vi "catch.vi"(8 "error out":errorcluster, 11 "KNR out":T2) -> (0 "error out 2":errorcluster, 1 "Circles (Shape Detection 1)":T1(array[cluster]) {"Position"."Y" format="%.2f"; "Position"."X" format="%.2f"}, 2 "Number of Matches (Shape Detection 1)":i32, 3 "KNR out 2":T2, 10 "X":dbl)   [LabVIEW 2013]
uses:
  <userlib>/KNR OS 3.0 LabVIEW Toolkit/Type Definition/KNR3 Reference.ctl
  <userlib>/_FPGA Interface Advanced Tools/FPGA Interface Base/FPGA Interface Base.lvclass
  <userlib>/KNR OS 3.0 LabVIEW Toolkit/Type Definition/Resource.ctl
panel:
  out "Voltage":dbl
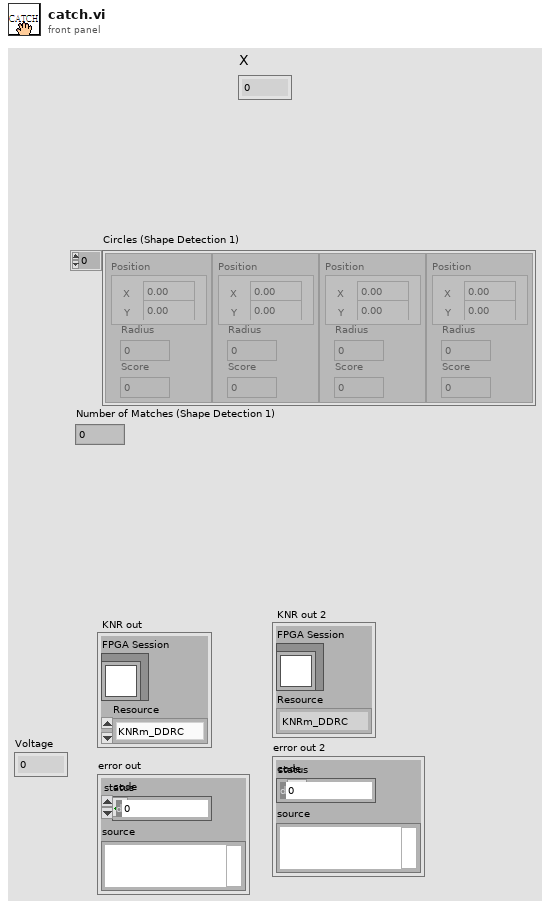
[diagram p1: front panel]
types:
  T1 = cluster{"Position":cluster{"X":sgl, "Y":sgl}, "Radius":dbl, "Score":dbl}[]
  T2 = typedef "KNR3 Reference.ctl" = cluster{"FPGA Session":refnum<class "FPGA Interface Base.lvclass">, "Resource":T3}
  T3 = typedef "Resource.ctl" = enum16{"KNRm_DDRC", "KNRm_DDDD", "KNRm_DDDR", "KNRm_DDDC", "KNR"}
  T4 = cluster{"Mode":enum16{"FRWD", "TURFIX", "TURNOF", "CIRCULAR"}, "Dir":enum16{"Left", "Right"}, "Pcmd":dbl, "Vcmd":dbl, "X":dbl, "Y":dbl}
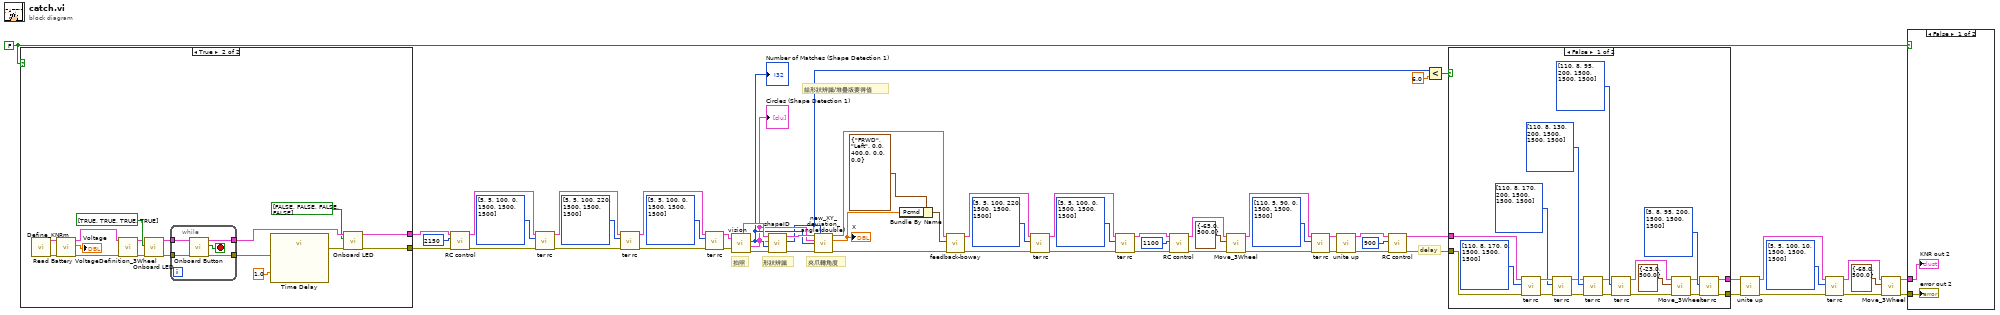
[diagram p0: block diagram]
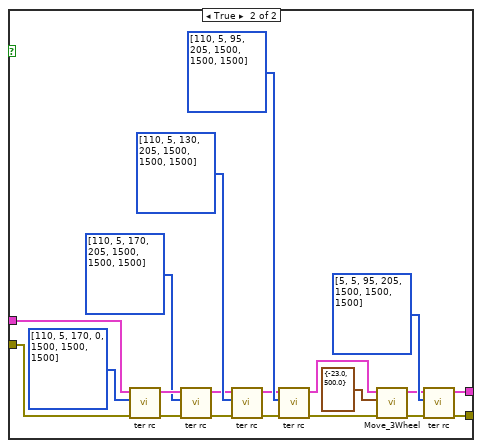
[diagram p2: hidden frame]
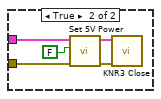
[diagram p3: hidden frame]
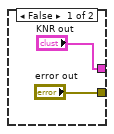
[diagram p4: hidden frame]
diagram:
  w61 = FALSE
  # "夾爪轉角度"
  # "形狀辨識"
  # "給形狀辨識/堆疊版要得值"
  # "拍照"
  # "delay"
  n1 = case shown="True" w61 {
    tunnel: ["KNR out" w69] -> w27
    tunnel: ["error out" w68] -> w26
    frame False {
    }
    frame True {
      n2 = call "Define_KNRm.vi"() -> ("error out"=w73:errorcluster, "KNR out"=w72:T2)  [unwired: 10 in]
      n3 = call <userlib>:"Read Battery Voltage.vi"("error in (no error)"=w73, "KNR in"=w72) -> ("error out"=w66:errorcluster, "Voltage"=→"Voltage":dbl, "KNR out"=w67:T2)  [unwired: 7 in]
      n4 = call "Definition_3Wheel.vi"("error in (no error)"=w66, "KNR in"=w67) -> ("error out"=w64:errorcluster, "KNR out"=w65:T2)  [unwired: 8 in]
      n5 = call <userlib>:"Onboard LED.vi"("error in (no error)"=w64, "LED List"=bool[] [TRUE, TRUE, TRUE, TRUE], "KNR in"=w65) -> ("error out"=w79:errorcluster, "KNR out"=w80:T2)  [unwired: 7 in]
      n6 = while {
        tunnel: w80 -> [w84]
        tunnel: w79 -> [w83]
        tunnel: [w82] -> w78
        tunnel: [w81] -> w76
        stop <- w85 stop-if-true
        n7 = call <userlib>:"Onboard Button.vi"("error in (no error)"=w83, "KNR in"=w84) -> ("error out"=w81:errorcluster, "value"=w85:bool, "KNR out"=w82:T2)  [unwired: 7 in]
      }
      n8 = call "Time Delay"("error in (no error)"=w76, "Delay Time (s)"=1.0) -> ("error out"=w75:errorcluster)  [unwired: 9 in]
      n9 = call <userlib>:"Onboard LED.vi"("error in (no error)"=w75, "LED List"=bool[] [FALSE, FALSE, FALSE, FALSE], "KNR in"=w78) -> ("error out"=w68:errorcluster, "KNR out"=w69:T2)  [unwired: 7 in]
    }
  }
  n10 = call "RC control.vi"("error in (no error)"=w26, "position"=2150, "KNR in"=w27) -> ("error out"=w50:errorcluster, "KNR out"=w51:T2)  [unwired: 7 in]
  n11 = call "ter rc.vi"("error in 2"=w50, "RC"=u16[] [5, 5, 100, 0, 1500, 1500, 1500], "KNR in 3"=w51) -> ("error out 4"=w34:errorcluster, "KNR out 4"=w35:T2)  [unwired: 7 in]
  n12 = call "ter rc.vi"("error in 2"=w34, "RC"=u16[] [5, 5, 100, 220, 1500, 1500, 1500], "KNR in 3"=w35) -> ("error out 4"=w23:errorcluster, "KNR out 4"=w47:T2)  [unwired: 7 in]
  n13 = call "ter rc.vi"("error in 2"=w23, "RC"=u16[] [5, 5, 100, 0, 1500, 1500, 1500], "KNR in 3"=w47) -> ("error out 4"=w55:errorcluster, "KNR out 4"=w56:T2)  [unwired: 7 in]
  n14 = call "vision.vi"("KNR in"=w56, "Error"=w55) -> ("KNR out"=w19:T2, "Number of Matches (Shape Detection 1)"=w15:i32, "Circles (Shape Detection 1)"=w14:T1, "error out"=w18:errorcluster)  [unwired: 1 in, 1 out]
  "Circles (Shape Detection 1)" <- w14
  "Number of Matches (Shape Detection 1)" <- w15
  n15 = call "shapeID.vi"("Error"=w18, "Nb Circles (Circle Detection 1)"=w15, "Circles (Shape Detection 1)"=w14, "KNR in"=w19) -> ("error out 4"=w16:errorcluster, "配對數"=w1:i32, "KNR out"=w17:T2)  [unwired: 4 in, 1 out]
  n16 = call "new_XY_deviation_angle(double).vi"("KNR in"=w17, "配對數"=w1, "Circles (Shape Detection 1)"=w14, "ふ计"=w15, "Error"=w16) -> ("KNR out"=w6:T2, "X"=w12:dbl, "error out"=w5:errorcluster)  [unwired: 6 in, 2 out]
  "X" <- w12
  n17 = Bundle By Name(cluster=T4 {"Mode"=enum."FRWD", "Dir"=enum."Left", "Pcmd"=0.0, "Vcmd"=400.0, "X"=0.0, "Y"=0.0} ("Move"), "Pcmd"=w12) -> (w11:T4)
  n18 = call "feedback-boway.vi"("error in (no error)"=w5, "Move"=w11, "KNR in"=w6) -> ("error out"=w42:errorcluster, "KNR out"=w43:T2)  [unwired: 6 in, 1 out]
  n19 = call "ter rc.vi"("error in 2"=w42, "RC"=u16[] [5, 5, 100, 220, 1500, 1500, 1500], "KNR in 3"=w43) -> ("error out 4"=w22:errorcluster, "KNR out 4"=w44:T2)  [unwired: 7 in]
  n20 = call "ter rc.vi"("error in 2"=w22, "RC"=u16[] [5, 5, 100, 0, 1500, 1500, 1500], "KNR in 3"=w44) -> ("error out 4"=w40:errorcluster, "KNR out 4"=w41:T2)  [unwired: 7 in]
  n21 = call "RC control.vi"("error in (no error)"=w40, "position"=1100, "KNR in"=w41) -> ("error out"=w3:errorcluster, "KNR out"=w4:T2)  [unwired: 7 in]
  n22 = call "Move_3Wheel.vi"("error in (no error)"=w3, "Cluster"=cluster{"UDmm)":dbl, "Vcmd":dbl} {"UDmm)"=-65.0, "Vcmd"=500.0}, "KNR in"=w4) -> ("error out"=w20:errorcluster, "KNR out"=w21:T2)  [unwired: 7 in]
  n23 = call "ter rc.vi"("error in 2"=w20, "RC"=u16[] [110, 5, 90, 0, 1500, 1500, 1500], "KNR in 3"=w21) -> ("error out 4"=w32:errorcluster, "KNR out 4"=w33:T2)  [unwired: 7 in]
  n24 = call "unite up.vi"("error in (no error)"=w32, "KNR in"=w33) -> ("error out"=w30:errorcluster, "KNR out"=w31:T2)  [unwired: 8 in]
  n25 = call "RC control.vi"("error in (no error)"=w30, "position"=900, "KNR in"=w31) -> ("error out"=w2:errorcluster, "KNR out"=w48:T2)  [unwired: 7 in]
  n26 = Less?(x=w1, y=6.0) -> (x < y?=w9:bool)
  n27 = case shown="False" w9 {
    tunnel: w2 -> [w94 w125]
    tunnel: w48 -> [w95 w124]
    tunnel: [w89 w109] -> w8
    tunnel: [w88 w108] -> w7
    frame False {
      n28 = call "ter rc.vi"("error in 2"=w94, "RC"=u16[] [110, 8, 170, 0, 1500, 1500, 1500], "KNR in 3"=w95) -> ("error out 4"=w104:errorcluster, "KNR out 4"=w103:T2)  [unwired: 7 in]
      n29 = call "ter rc.vi"("error in 2"=w104, "RC"=u16[] [110, 8, 170, 200, 1500, 1500, 1500], "KNR in 3"=w103) -> ("error out 4"=w99:errorcluster, "KNR out 4"=w100:T2)  [unwired: 7 in]
      n30 = call "ter rc.vi"("error in 2"=w99, "RC"=u16[] [110, 8, 130, 200, 1500, 1500, 1500], "KNR in 3"=w100) -> ("error out 4"=w96:errorcluster, "KNR out 4"=w97:T2)  [unwired: 7 in]
      n31 = call "ter rc.vi"("error in 2"=w96, "RC"=u16[] [110, 8, 95, 200, 1500, 1500, 1500], "KNR in 3"=w97) -> ("error out 4"=w86:errorcluster, "KNR out 4"=w87:T2)  [unwired: 7 in]
      n32 = call "Move_3Wheel.vi"("error in (no error)"=w86, "Cluster"=cluster{"UDmm)":dbl, "Vcmd":dbl} {"UDmm)"=-23.0, "Vcmd"=500.0}, "KNR in"=w87) -> ("error out"=w90:errorcluster, "KNR out"=w91:T2)  [unwired: 7 in]
      n33 = call "ter rc.vi"("error in 2"=w90, "RC"=u16[] [5, 8, 95, 200, 1500, 1500, 1500], "KNR in 3"=w91) -> ("error out 4"=w88:errorcluster, "KNR out 4"=w89:T2)  [unwired: 7 in]
    }
    frame True {
      n34 = call "ter rc.vi"("error in 2"=w125, "RC"=u16[] [110, 5, 170, 0, 1500, 1500, 1500], "KNR in 3"=w124) -> ("error out 4"=w122:errorcluster, "KNR out 4"=w121:T2)  [unwired: 7 in]
      n35 = call "ter rc.vi"("error in 2"=w122, "RC"=u16[] [110, 5, 170, 205, 1500, 1500, 1500], "KNR in 3"=w121) -> ("error out 4"=w117:errorcluster, "KNR out 4"=w118:T2)  [unwired: 7 in]
      n36 = call "ter rc.vi"("error in 2"=w117, "RC"=u16[] [110, 5, 130, 205, 1500, 1500, 1500], "KNR in 3"=w118) -> ("error out 4"=w114:errorcluster, "KNR out 4"=w115:T2)  [unwired: 7 in]
      n37 = call "ter rc.vi"("error in 2"=w114, "RC"=u16[] [110, 5, 95, 205, 1500, 1500, 1500], "KNR in 3"=w115) -> ("error out 4"=w106:errorcluster, "KNR out 4"=w107:T2)  [unwired: 7 in]
      n38 = call "Move_3Wheel.vi"("error in (no error)"=w106, "Cluster"=cluster{"UDmm)":dbl, "Vcmd":dbl} {"UDmm)"=-23.0, "Vcmd"=500.0}, "KNR in"=w107) -> ("error out"=w110:errorcluster, "KNR out"=w111:T2)  [unwired: 7 in]
      n39 = call "ter rc.vi"("error in 2"=w110, "RC"=u16[] [5, 5, 95, 205, 1500, 1500, 1500], "KNR in 3"=w111) -> ("error out 4"=w108:errorcluster, "KNR out 4"=w109:T2)  [unwired: 7 in]
    }
  }
  n40 = call "unite up.vi"("error in (no error)"=w7, "KNR in"=w8) -> ("error out"=w28:errorcluster, "KNR out"=w29:T2)  [unwired: 8 in]
  n41 = call "ter rc.vi"("error in 2"=w28, "RC"=u16[] [5, 5, 100, 10, 1500, 1500, 1500], "KNR in 3"=w29) -> ("error out 4"=w37:errorcluster, "KNR out 4"=w38:T2)  [unwired: 7 in]
  n42 = call "Move_3Wheel.vi"("error in (no error)"=w37, "Cluster"=cluster{"UDmm)":dbl, "Vcmd":dbl} {"UDmm)"=-68.0, "Vcmd"=500.0}, "KNR in"=w38) -> ("error out"=w24:errorcluster, "KNR out"=w25:T2)  [unwired: 7 in]
  n43 = case shown="False" w61 {
    tunnel: w25 -> [w127 w129]
    tunnel: w24 -> [w126 w128]
    frame False {
      "error out 2" <- w126
      "KNR out 2" <- w127
    }
    frame True {
      n44 = call <userlib>:"Set 5V Power.vi"("error in (no error)"=w128, "5V Power(T)"=FALSE, "KNR in"=w129) -> ("error out"=w131:errorcluster, "KNR out"=w132:T2)  [unwired: 7 in]
      n45 = call <userlib>:"KNR3 Close.vi"("error in (no error)"=w131, "KNR in"=w132) -> ()  [unwired: 9 in, 1 out]
    }
  }
